vi "消噪结果.vi"() -> (0 "端点检测的结束帧":dbl format="%.2f", 1 "端点检测的起始帧":dbl format="%.2f", 2 "限制幅度后的语音信号":dbl[](graph), 3 "各帧的ef(n)值":dbl[][](graph), 4 "干净语音段":dbl[](graph), 5 "预加重后的语音信号":dbl[](graph), 6 "消噪后的语音信号":dbl[](graph), 7 "Waveform Graph 2":i16[](graph))   [LabVIEW 2013]
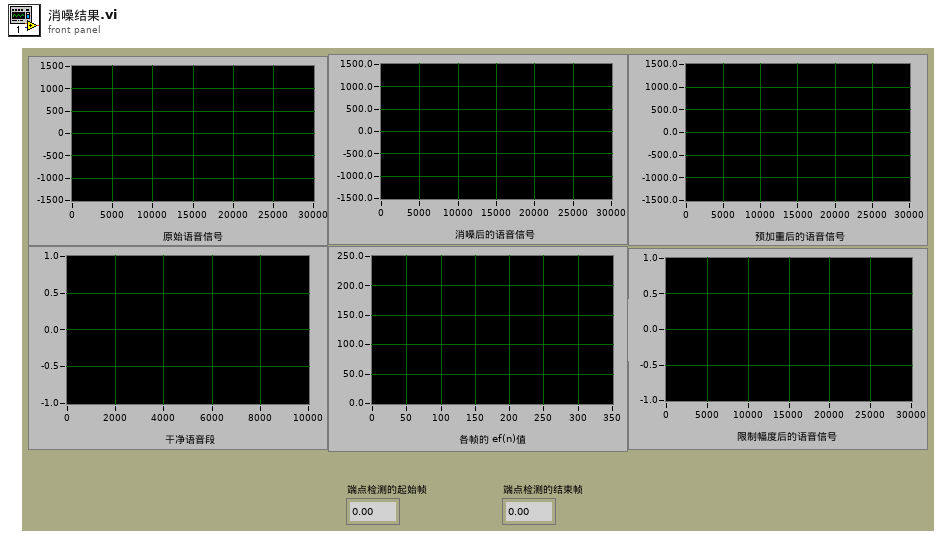
[diagram p1: front panel]
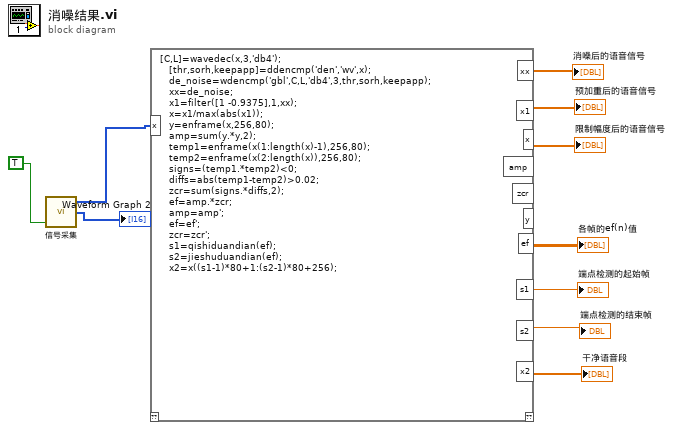
[diagram p0: block diagram]
diagram:
  n1 = call "信号采集.vi"("Boolean"=TRUE) -> ("mono 16-bit"=→"Waveform Graph 2":i16[], "波形图"=w2:i16[])
  n2 = script code="[C,L]=wavedec(x,3,'db4');\n   [thr,sorh,keepapp]=ddencmp('den','wv',x);\n   de_noise=wdencmp('gbl',C,L,'db4',3,thr,sorh,keepapp);\n   xx=de_noise;\n   x1=filter([1 -0.9375],1,xx);\n   x=x1/max(abs(x1));\n   y=enframe(x,256,80);\n   amp=sum(y.*y,2);\n   temp1=enframe(x(1:length(x)-1),256,80);\n   temp2=enframe(x(2:length(x)),256,80);\n   signs=(temp1.*temp2)<0;\n   diffs=abs(temp1-temp2)>0.02;\n   zcr=sum(signs.*diffs,2);\n   ef=amp.*zcr;\n   amp=amp';\n   ef=ef';\n   zcr=zcr';\n   s1=qishiduandian(ef);\n   s2=jieshuduandian(ef);\n   x2=x((s1-1)*80+1:(s2-1)*80+256);"("x"=w2) -> ("xx"=→"消噪后的语音信号":dbl[], "x1"=→"预加重后的语音信号":dbl[], "x"=→"限制幅度后的语音信号":dbl[], "ef"=→"各帧的ef(n)值":dbl[][], "s1"=→"端点检测的起始帧":dbl, "s2"=→"端点检测的结束帧":dbl, "x2"=→"干净语音段":dbl[])  [unwired: 1 in, 4 out]
